vi "StopUIProgress.vi"(8 "error in (no error)":errorcluster, 11 "Progress in":refnum<class "Progress.lvclass">) -> (0 "error out":errorcluster, 3 "Progress out":refnum<class "Progress.lvclass">)   [LabVIEW 2020, in "Progress.lvlib" / "Progress.lvclass"]
uses:
  Progress.lvclass
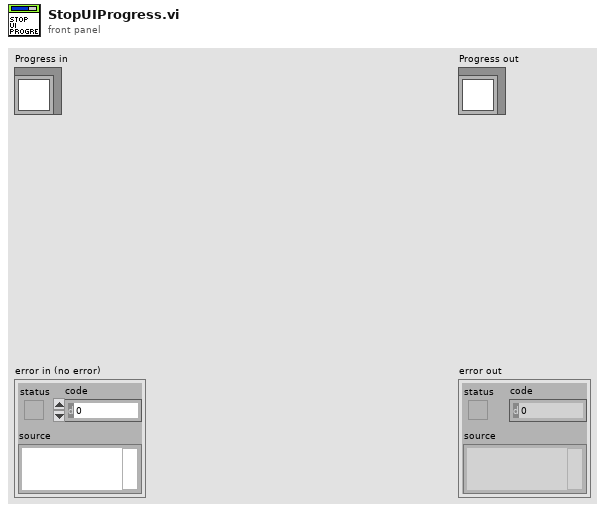
[diagram p1: front panel]
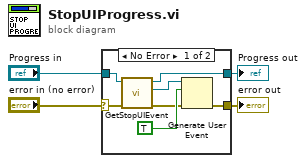
[diagram p0: block diagram]
diagram:
  n1 = case shown="No Error" "error in (no error)" {
    selector: "error in (no error)" -> [w7 w13]
    tunnel: [w5 w13] -> w3
    tunnel: [w11 w12] -> w1
    tunnel: "Progress in" -> [w10 w12]
    frame No Error {
      n2 = call "GetStopUIEvent.vi"("error in (no error)"=w7, "Progress in"=w10) -> ("error out"=w6:errorcluster, "StopUIEvent"=w9:refnum<user-event>, "Progress out"=w11:refnum<class "Progress.lvclass">)  [unwired: 7 in]
      n3 = Generate User Event(user event=w9, event data cluster=TRUE ("event data"), error in=w6) -> (error out=w5:errorcluster)  [unwired: 1 in, 1 out]
    }
    frame Error {
    }
  }
  "error out" <- w3
  "Progress out" <- w1
